vi "Error Cluster From Error Code.vi"(4 "is warning? (False)":bool, 5 "show call chain? (False)":bool, 6 "error in (no error)":errorcluster, 7 "Call Depth":i32, 8 "error message (\"\")":string, 9 "error code (0)":i32) -> (0 "error out":errorcluster)   [LabVIEW 2017, in "JSONtext.lvlib"]
doc: "Converts an error or warning code to an error cluster. This VI is useful when you receive a return value from a shared library call or when you return user-defined error codes."
uses:
  JSONtext.lvlib
panel:
  in  "call chain header":string="\n<b>Complete call chain:</b>"
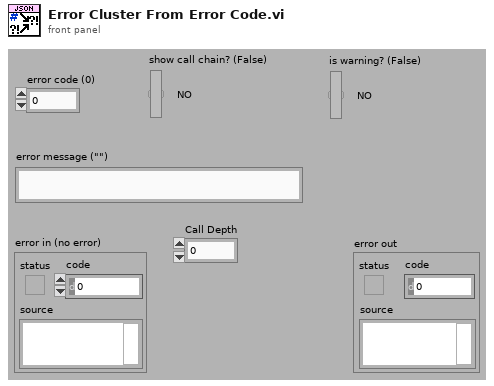
[diagram p1: front panel]
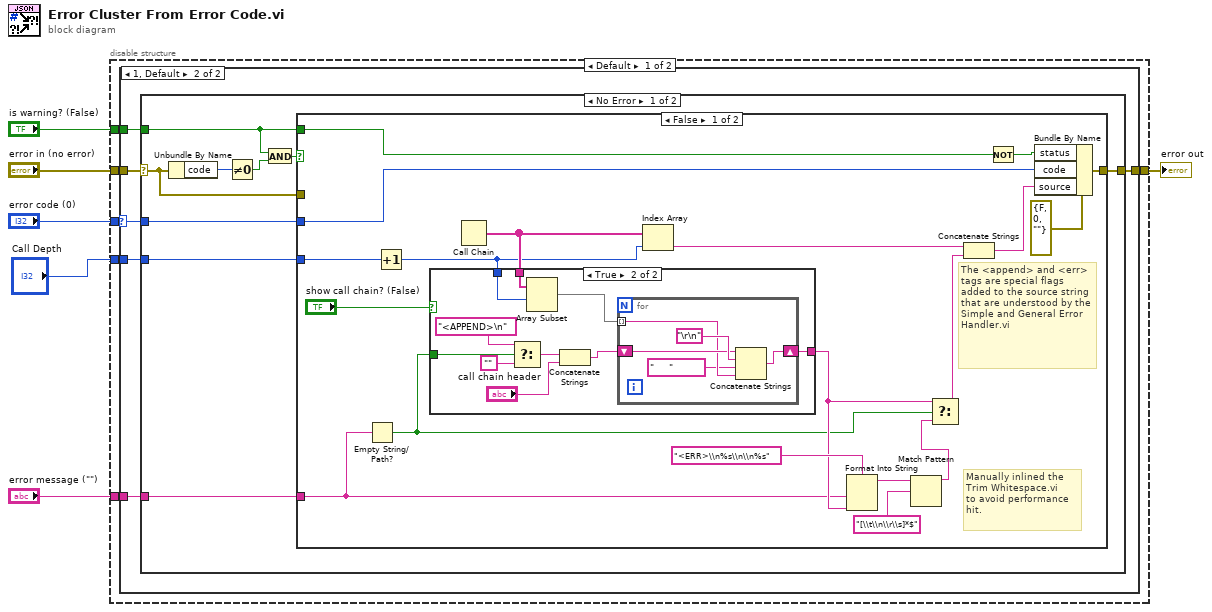
[diagram p0: block diagram]
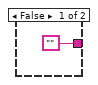
[diagram p3: hidden frame]
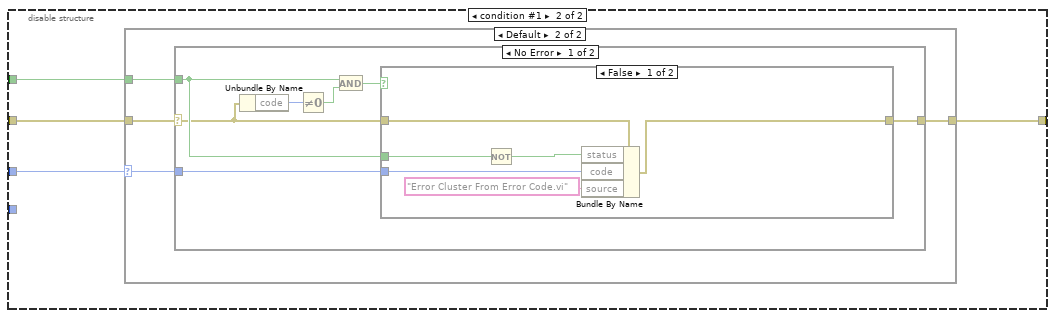
[diagram p6: hidden frame]
diagram:
  n1 = disable-structure shown="Default" {
    disable-tunnel: [w12 w68] -> w6
    disable-tunnel: "error in (no error)" -> [w11 w69]
    disable-tunnel: "error code (0)" -> [w10 w67]
    disable-tunnel: "error message (\"\")" -> [w9 _]
    disable-tunnel: "is warning? (False)" -> [w8 w66]
    disable-tunnel: "Call Depth" -> [w7 _]
    frame condition #0 (active) {
      n2 = case shown="1, Default" w10 {
        selector: w10 -> [_ w17]
        tunnel: [w13 w19] -> w12
        tunnel: w11 -> [w13 w18]
        tunnel: w9 -> [_ w16]
        tunnel: w8 -> [_ w15]
        tunnel: w7 -> [_ w14]
        frame 0 {
          # "If the error code in equals zero, then propagate the error in cluster regardless of its value."
        }
        frame 1, Default {
          n3 = case shown="No Error" w18 {
            selector: w18 -> [w23 w65]
            tunnel: [w28 w65] -> w19
            tunnel: w17 -> [w27 _]
            tunnel: w16 -> [w22 _]
            tunnel: w15 -> [w21 _]
            tunnel: w14 -> [w20 _]
            frame No Error {
              n4 = Unbundle By Name(w23) -> ("code"=w26:i32)
              n5 = Not Equal To 0?(x=w26) -> (x != 0?=w24:bool)
              n6 = And(x=w21, y=w24) -> (x .and. y?=w25:bool)
              n7 = case shown="False" w25 {
                tunnel: [w47 w64] -> w28
                tunnel: w27 -> [w43 _]
                tunnel: w23 -> [_ w64]
                tunnel: w21 -> [w41 _]
                tunnel: w22 -> [w36 _]
                tunnel: w20 -> [w30 _]
                frame False {
                  # "Manually inlined the\nTrim Whitespace.vi\nto avoid performance\nhit."
                  # "The <append> and <err> tags are special flags added to the source string that are understood by the Simple and General Error Handler.vi"
                  n8 = Empty String/Path?(string/path=w36) -> (empty?=w35:bool)
                  n9 = Increment(x=w30) -> (x+1=w29:i32)
                  n10 = Call Chain() -> (call chain=w42:string[])
                  n11 = case shown="True" "show call chain? (False)" {
                    tunnel: ["" w58] -> w38
                    tunnel: w42 -> [_ w57]
                    tunnel: w35 -> [_ w53]
                    tunnel: w29 -> [_ w49]
                    frame False {
                    }
                    frame True {
                      n12 = Select(t="<APPEND>\n", s=w53, f="") -> (s? t:f=w50:string)
                      n13 = Array Subset(array=w57, index=w49) -> (w56:string[])  [unwired: 1 in]
                      n14 = Concatenate Strings(w50, "call chain header") -> (w54:string)
                      n15 = for {
                        tunnel: w56 -> [w60] mode=indexing
                        shift-right: [w63] -> w58
                        shift-left: w54 -> [w61]
                        n16 = Concatenate Strings(w61, "\r\n", "     ", w60) -> (w63:string)
                      }
                    }
                  }
                  n17 = Index Array(array=w42, index=w29) -> (element=w31:string)
                  n18 = Format Into String(format string="<ERR>\\n%s\\n\\n%s", w36, w38) -> (resulting string=w33:string)  [unwired: 2 in, 1 out]
                  n19 = Match Pattern(string=w33, regular expression="[\\t\\n\\r\\s]*$") -> (before substring=w32:string)  [unwired: 1 in, 3 out]
                  n20 = Select(t=w38, s=w35, f=w32) -> (s? t:f=w37:string)
                  n21 = Concatenate Strings(w31, w37) -> (w45:string)
                  n22 = Not(x=w41) -> (.not. x?=w44:bool)
                  n23 = Bundle By Name(cluster=errorcluster {"status"=FALSE, "code"=0, "source"=""} ("error out"), "status"=w44, "code"=w43, "source"=w45) -> (w47:errorcluster)
                }
                frame True {
                  # "If the error code input is setting a warning, and a warning is already set on the wire, then we\ngo with the one already on the wire."
                }
              }
            }
            frame Error {
              # "An error in trumps any error code input."
            }
          }
        }
      }
    }
    frame condition #1 {
      n24 = case shown="Default" w67 {
        selector: w67 -> [_ w72]
        tunnel: w69 -> [w70 w74]
        tunnel: [w70 w73] -> w68
        tunnel: w66 -> [_ w71]
        frame 0 {
          # "If the error code in equals zero, then propagate the error in cluster regardless of its value."
        }
        frame Default {
          n25 = case shown="No Error" w74 {
            selector: w74 -> [w76 w89]
            tunnel: [w80 w89] -> w73
            tunnel: w72 -> [w81 _]
            tunnel: w71 -> [w77 _]
            frame No Error {
              n26 = Unbundle By Name(w76) -> ("code"=w79:i32)
              n27 = Not Equal To 0?(x=w79) -> (x != 0?=w78:bool)
              n28 = And(x=w77, y=w78) -> (x .and. y?=w75:bool)
              n29 = case shown="False" w75 {
                tunnel: w81 -> [w87 _]
                tunnel: [w84 w88] -> w80
                tunnel: w77 -> [w83 _]
                tunnel: w76 -> [w82 w88]
                frame False {
                  n30 = Not(x=w83) -> (.not. x?=w86:bool)
                  n31 = Bundle By Name(cluster=w82, "status"=w86, "code"=w87, "source"="Error Cluster From Error Code.vi") -> (w84:errorcluster)
                }
                frame True {
                  # "If the error code input is setting a warning, and a warning is already set on the wire, then we\ngo with the one already on the wire."
                }
              }
            }
            frame Error {
              # "An error in trumps any error code input."
            }
          }
        }
      }
    }
  }
  "error out" <- w6
